vi "Read_LegProperties.vi"(8 "error in (no error)":errorcluster, 11 "CAlex2 in":refnum<class "CAlex2.lvclass">) -> (0 "error out":errorcluster, 2 "LegProperties":T1, 3 "CAlex2 out":refnum<class "CAlex2.lvclass">)   [LabVIEW 2015, in "CAlex2.lvclass"]
uses:
  CAlex2.lvclass
  TypeDef/LowerBodyDim.ctl
  CAlex2.lvclass/CAlex2.ctl
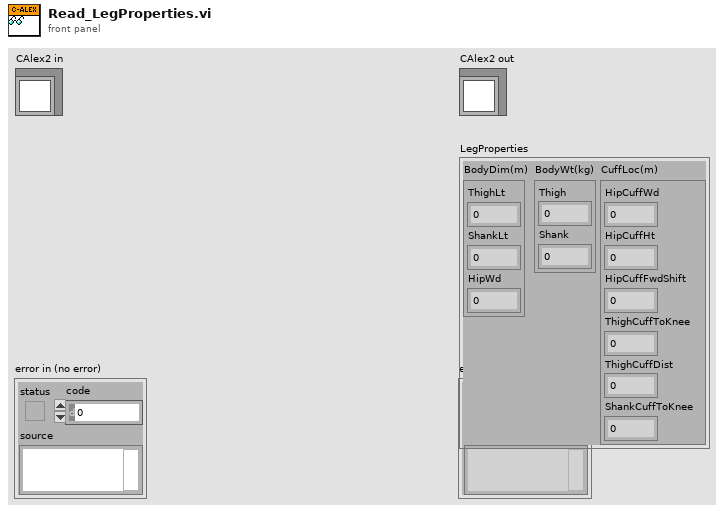
[diagram p1: front panel]
types:
  T1 = typedef "CAlex2.lvclass/LowerBodyDim.ctl" = cluster{"BodyDim(m)":cluster{"ThighLt":dbl, "ShankLt":dbl, "HipWd":dbl}, "BodyWt(kg)":cluster{"Thigh":dbl, "Shank":dbl}, "CuffLoc(m)":cluster{"HipCuffWd":dbl, "HipCuffHt":dbl, "HipCuffFwdShift":dbl, "ThighCuffToKnee":dbl, "ThighCuffDist":dbl, "ShankCuffToKnee":dbl}}
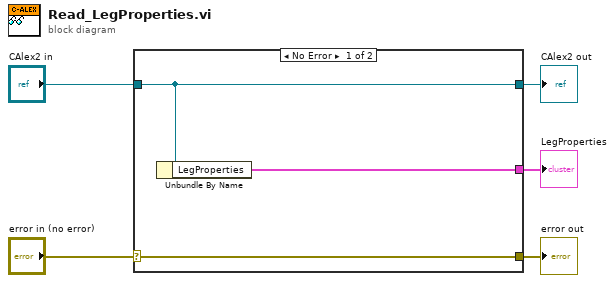
[diagram p0: block diagram]
diagram:
  n1 = case shown="No Error" "error in (no error)" {
    selector: "error in (no error)" -> [w8 w9]
    tunnel: [w8 w9] -> w4
    tunnel: [w7 w10] -> w2
    tunnel: "CAlex2 in" -> [w7 w10]
    tunnel: [w6 _] -> w1
    frame No Error {
      n2 = Unbundle By Name(w7) -> ("LegProperties"=w6:T1)
    }
    frame Error {
    }
  }
  "error out" <- w4
  "CAlex2 out" <- w2
  "LegProperties" <- w1
